vi "set call chain.vi"(11 "exception in":T1 {"code" format="%.0x"}) -> (3 "exception out":T1 {"code" format="%.0x"})   [LabVIEW 2013, in "exception.lvlib"]
uses:
  exception.lvlib
  exception.ctl
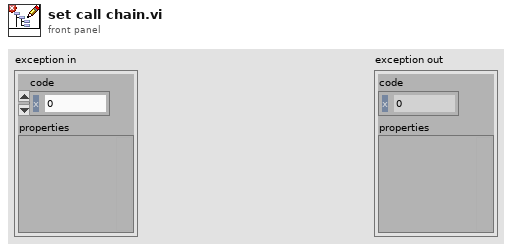
[diagram p1: front panel]
types:
  T1 = typedef "exception.lvlib/exception.ctl" = cluster{"code":i32, "properties":variant}
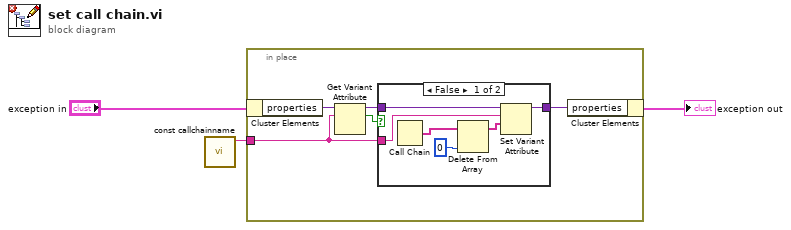
[diagram p0: block diagram]
diagram:
  n1 = call "const callchainname.vi"() -> ("label"=w1:string)  [unwired: 11 in]
  n2 = in-place {
    in-place-border: w1 -> [w7]
    n3 = in-place-cluster #1("exception in") -> ("properties"=w6:variant)
    n4 = Get Variant Attribute(Variant=w6, name=w7) -> (duplicate Variant=w5:variant, found=w4:bool)  [unwired: 2 in, 2 out]
    n5 = case shown="False" w4 {
      tunnel: w5 -> [w14 w15]
      tunnel: [w13 w15] -> w8
      tunnel: w7 -> [w12 _]
      frame False {
        n6 = Call Chain() -> (call chain=w10:string[])
        n7 = Delete From Array(array=w10, index=0) -> (array with subset deleted=w9:string[])  [unwired: 1 in, 1 out]
        n8 = Set Variant Attribute(Variant=w14, name=w12, value=w9) -> (Variant out=w13:variant)  [unwired: 1 in, 2 out]
      }
      frame True {
      }
    }
    n9 = in-place-cluster #1("properties"=w8) -> (→"exception out":T1)
  }
